vi "Picture_dif_Save_to_matlab.vi"   [LabVIEW 2011]
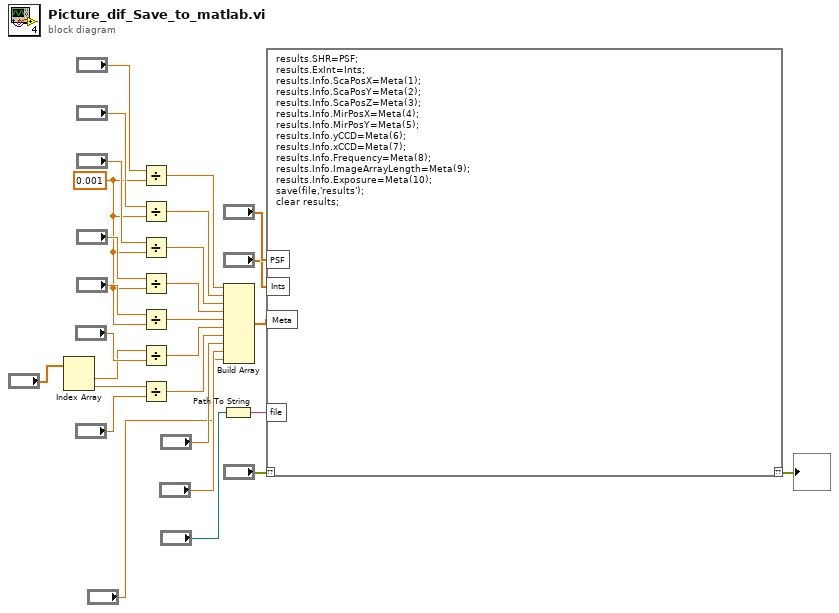
[diagram p0: block diagram]
diagram:
  w7 = 0.001 ("y")
  n1 = Index Array(array="?") -> (element #1=w4:dbl, element #2=w3:dbl)  [unwired: 2 in]
  n2 = Divide(x="?", y=w7) -> (x/y=w20:dbl)
  n3 = Divide(x="?", y=w7) -> (x/y=w19:dbl)
  n4 = Divide(x="?", y=w7) -> (x/y=w22:dbl)
  n5 = Divide(x="?", y=w7) -> (x/y=w21:dbl)
  n6 = Divide(x="?", y=w7) -> (x/y=w23:dbl)
  n7 = Divide(x=w4, y="?") -> (x/y=w24:dbl)
  n8 = Divide(x=w3, y="?") -> (x/y=w25:dbl)
  n9 = Path To String(path="?") -> (string=w27:string)
  n10 = Build Array(w20, w19, w22, w21, w23, w24, w25, "?", "?", "?") -> (w26:dbl[])
  n11 = script code="results.SHR=PSF;\nresults.ExInt=Ints;\nresults.Info.ScaPosX=Meta(1);\nresults.Info.ScaPosY=Meta(2);\nresults.Info.ScaPosZ=Meta(3);\nresults.Info.MirPosX=Meta(4);\nresults.Info.MirPosY=Meta(5);\nresults.Info.yCCD=Meta(6);\nresults.Info.xCCD=Meta(7);\nresults.Info.Frequency=Meta(8);\nresults.Info.ImageArrayLength=Meta(9);\nresults.Info.Exposure=Meta(10);\nsave(file,'results');\nclear results;"("??"="?", "PSF"="?", "Ints"="?", "Meta"=w26, "file"=w27) -> ("??"=→"?":errorcluster)
